vi "PV ASM340 Calibration.vi"(0 "VISA session":refnum<visa-resource-name>, 1 "Adress of unit":u16=1 min=1 max=999 step=1, 5 "Parameter":u16(ring) items=[" Calibration State (667)", " Leakrate external testleak vacuum (671)", " Leakrate external testleak sniff (673)", " Leakrate internal testleak (676)", " Calibration factor high (read only) (694)"], 7 "Parameter\nread only<->describe":bool, 11 "error in (no error)":errorcluster, 12 "Leakrate value in":dbl=1e-07 format="%.2e") -> (4 "dup VISA session":refnum<visa-resource-name>, 6 "response (data)":string, 10 "Calibration state out":i8(ring) items=["--", "Connect TL", "Pumping", "Measure TF high", "Massadjust", "Calibrate TF high", "Calibrate TF low", "Calibrate Counter Flow", "Remove TL", "Background TF high", "Background TF low", "Background Counter Flow", "Wait for confirmation"], 15 "error out":errorcluster)   [LabVIEW 2021, in "Pfeiffer Vacuum.lvlib"]
doc: "There are 5 parameters available, only one of which can be enabled at a time. \n\n0 - Calibration State (default) - Para 667\n1 - Leakrate external testleak vacuum - Para 671\n2 - Leakrate external testleak sniff - Para 673\n3 - Leakrate internal testleak - Para 676\n4 - Calibration factor high (read only) - Para 694\n\nNote: Any settings for an parameter that is not selected will be ignored. If a value is out of range, it will be changed to either the upper or the lower limit of the range."
uses:
  <instrlib>/Pfeiffer Vacuum/Pfeiffer Vacuum.lvlib
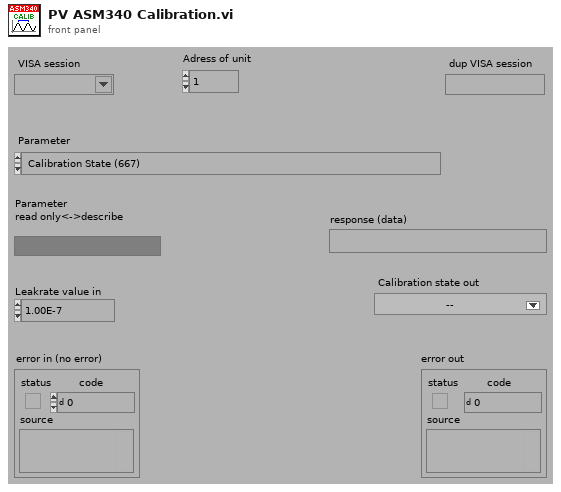
[diagram p1: front panel]
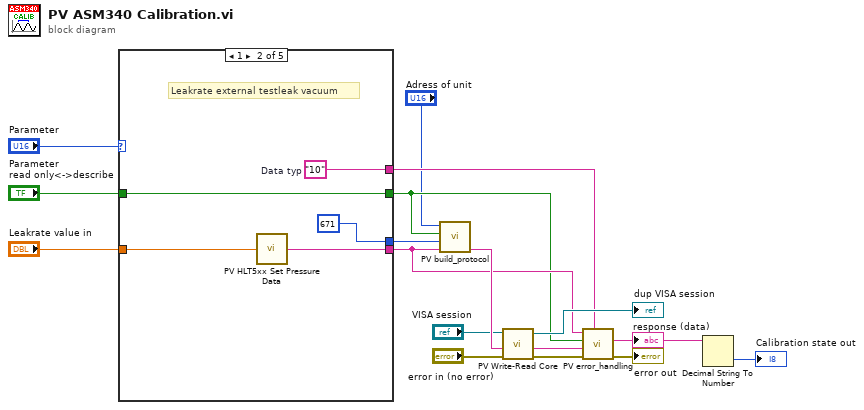
[diagram p0: block diagram]
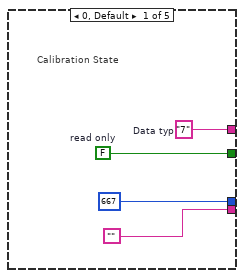
[diagram p2: hidden frame]
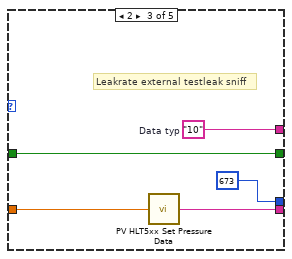
[diagram p3: hidden frame]
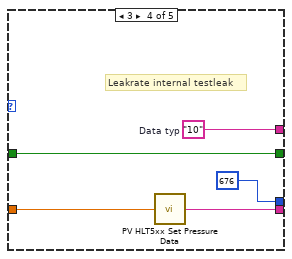
[diagram p4: hidden frame]
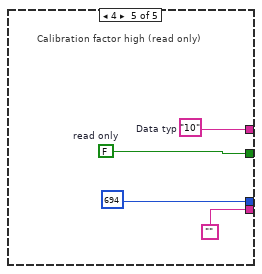
[diagram p5: hidden frame]
diagram:
  n1 = case shown="1" "Parameter" {
    tunnel: [u16 667 ("Parameter-number") u16 671 ("Parameter-number") u16 673 ("Parameter-number") u16 676 ("Parameter-number") u16 694 ("Parameter-number")] -> w17
    tunnel: ["" w22 w28 w32 ""] -> w12
    tunnel: [w20 w24 w30 w35 w39] -> w10
    tunnel: "Parameter\nread only<->describe" -> [_ w24 w30 w35 _]
    tunnel: [w21 w26 w31 w36 w40] -> w11
    tunnel: "Leakrate value in" -> [_ w23 w27 w33 _]
    frame 0, Default {
      w20 = FALSE  # read only
      w21 = "7"  # Data typ
      # "Calibration State"
    }
    frame 1 {
      w26 = "10"  # Data typ
      # "Leakrate external testleak vacuum"
      n2 = call <instrlib>:"PV HLT5xx Set Pressure Data.vi"("Value in"=w23) -> ("Output"=w22:string)
    }
    frame 2 {
      w31 = "10"  # Data typ
      # "Leakrate external testleak sniff"
      n3 = call <instrlib>:"PV HLT5xx Set Pressure Data.vi"("Value in"=w27) -> ("Output"=w28:string)
    }
    frame 3 {
      w36 = "10"  # Data typ
      # "Leakrate internal testleak"
      n4 = call <instrlib>:"PV HLT5xx Set Pressure Data.vi"("Value in"=w33) -> ("Output"=w32:string)
    }
    frame 4 {
      w39 = FALSE  # read only
      w40 = "10"  # Data typ
      # "Calibration factor high (read only)"
    }
  }
  n5 = call <instrlib>:"PV build_protocol.vi"("Data"=w12, "Parameter-number"=w17, "parameter\nread<->describe"=w10, "Adress"="Adress of unit") -> ("output"=w16:string)  [unwired: 3 in]
  n6 = call <instrlib>:"PV Write-Read Core.vi"("error in"="error in (no error)", "Write data in"=w16, "VISA session"="VISA session") -> ("error out"=w14:errorcluster, "response (data) out"=w15:string, "dup VISA session"=→"dup VISA session":refnum<visa-resource-name>)  [unwired: 2 in]
  n7 = call <instrlib>:"PV error_handling.vi"("Data Typ in"=w11, "error in"=w14, "response (data) in"=w15, "Parameter\nread only<->describe"=w10, "data in"=w12) -> ("error out"=→"error out":errorcluster, "Data out"=w8:string)  [unwired: 4 in, 1 out]
  "response (data)" <- w8
  n8 = Decimal String To Number(string=w8) -> (number=→"Calibration state out":i32)  [unwired: 2 in, 1 out]
